vi "Adjustmentlog.vi"(5 "Variant":string, 7 "nominalLevel":string, 8 "error in (no error)":errorcluster, 9 "Level":dbl[](array[numeric]), 10 "Amplitude":dbl[](array[numeric]), 11 "Frequencies":dbl[](array[numeric])) -> (0 "error IO":errorcluster)   [LabVIEW 2018]
panel:
  out "concatenated string":string caption="File Content"
  out "date/time string":string
  out "path":path
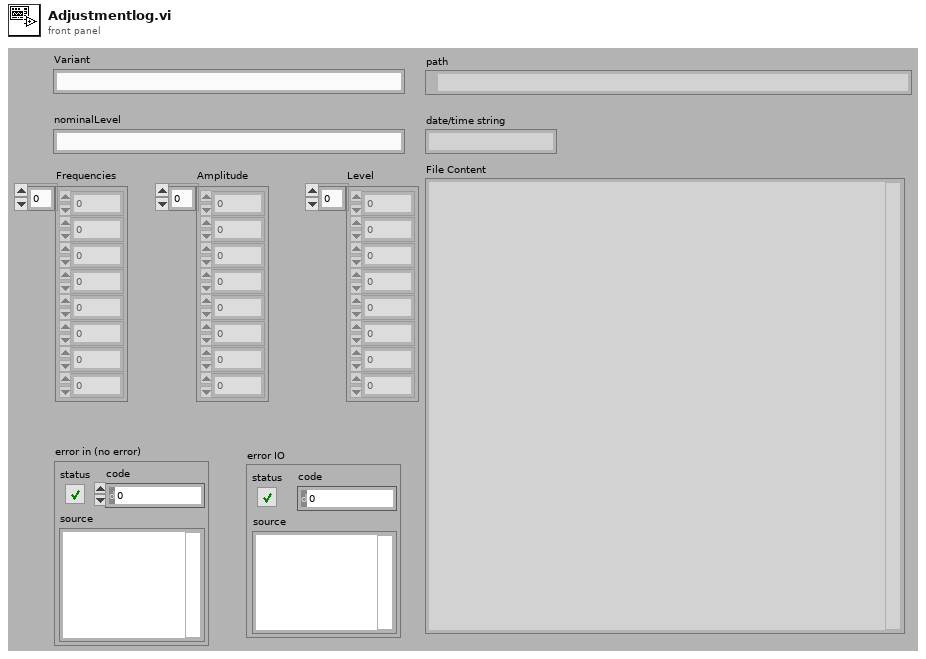
[diagram p1: front panel]
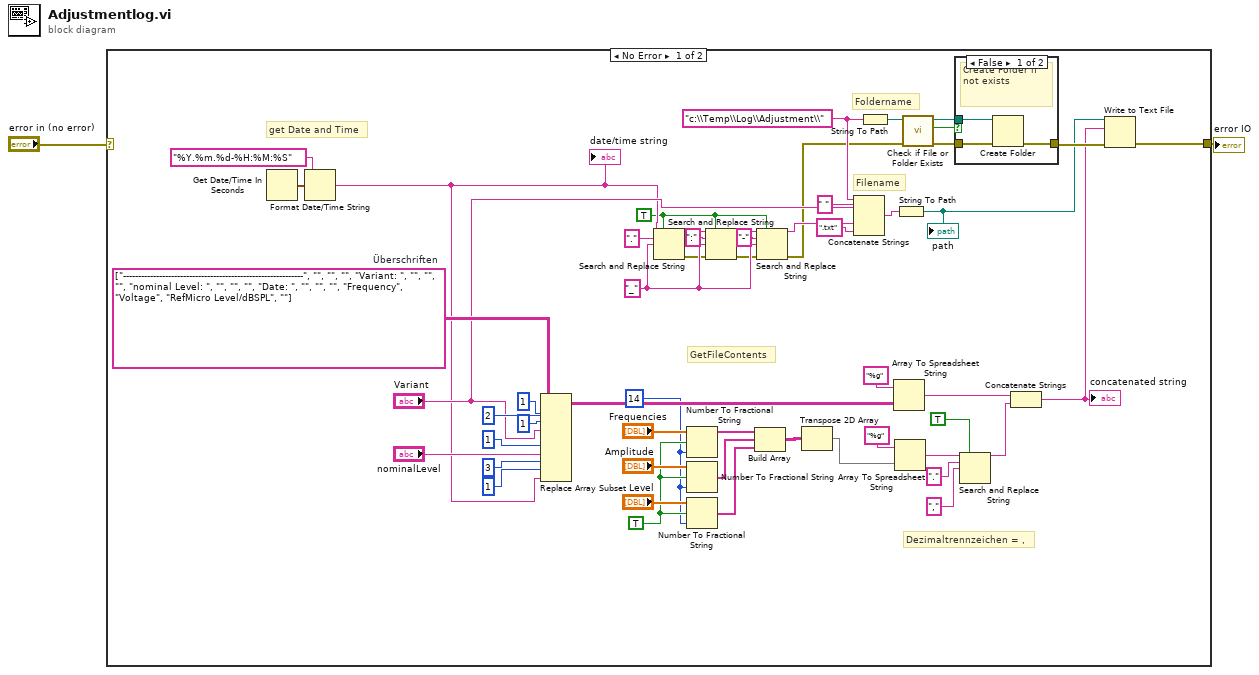
[diagram p0: block diagram]
diagram:
  n1 = case shown="No Error" "error in (no error)" {
    selector: "error in (no error)" -> [_ w61]
    tunnel: [w53 w61] -> w2
    frame No Error {
      w3 = i16 14 ("precision (6)")
      w5 = TRUE ("use system decimal point (T)")
      w34 = "_" ("replace string (\"\")")
      w31 = TRUE ("replace all? (F)")
      w25 = "c:\\Temp\\Log\\Adjustment\\" ("string")
      w46 = string[][] [["------------------------------------------------------------", "", "", ""], ["Variant: ", "", "", ""], ["nominal Level: ", "", "", ""], ["Date: ", "", "", ""], ["Frequency", "Voltage", "RefMicro Level/dBSPL", ""]]  # Überschriften
      # "Dezimaltrennzeichen = ,"
      # "get Date and Time"
      # "GetFileContents"
      # "Foldername"
      # "Filename"
      n2 = Get Date/Time In Seconds() -> (seconds since 1Jan1904=w43:timestamp)
      n3 = Format Date/Time String(time format string (%c)="%Y.%m.%d-%H:%M:%S", seconds (now)=w43) -> (date/time string=w38:string)  [unwired: 1 in]
      "date/time string" <- w38
      n4 = Replace Array Subset(array=w46, new element #1="Variant", index (row) #1=1 ("Index (Zeile)"), index (col) #1=1 ("Deaktivierter Index (Spalte)"), new element #2="nominalLevel", index (row) #2=2 ("Index (Zeile)"), index (col) #2=1 ("Deaktivierter Index (Spalte)"), new element #3=w38, index (row) #3=3 ("Index (Zeile)"), index (col) #3=1 ("Deaktivierter Index (Spalte)")) -> (w13:string[][])
      n5 = Search and Replace String(replace all?=w31, input string=w38, search string=".", replace string=w34) -> (result string=w36:string, error out=w22:errorcluster)  [unwired: 4 in, 2 out]
      n6 = Number To Fractional String(use system decimal point (T)=w5, number="Frequencies", precision (6)=w3) -> (F-format string=w19:string[])  [unwired: 1 in]
      n7 = Number To Fractional String(use system decimal point (T)=w5, number="Amplitude", precision (6)=w3) -> (F-format string=w54:string[])  [unwired: 1 in]
      n8 = Number To Fractional String(use system decimal point (T)=w5, number="Level", precision (6)=w3) -> (F-format string=w16:string[])  [unwired: 1 in]
      n9 = Search and Replace String(replace all?=w31, input string=w36, search string=":", replace string=w34, error in=w22) -> (result string=w35:string, error out=w21:errorcluster)  [unwired: 3 in, 2 out]
      n10 = Build Array(w19, w54, w16) -> (w45:string[][])
      n11 = Search and Replace String(replace all?=w31, input string=w35, search string="-", replace string=w34, error in=w21) -> (result string=w30:string, error out=w20:errorcluster)  [unwired: 3 in, 2 out]
      n12 = Transpose 2D Array(2D array=w45) -> (transposed array=w12:string[][])
      n13 = Concatenate Strings(w25, "Variant", " " ("string"), w30, ".txt" ("string")) -> (w39:string)
      n14 = String To Path(string=w25) -> (path=w24:path)
      n15 = Array To Spreadsheet String(array=w13, 3:"%g" ("Format-String")) -> (spreadsheet string=w6:string)  [unwired: 1 in]
      n16 = Array To Spreadsheet String(array=w12, 3:"%g" ("Format-String")) -> (spreadsheet string=w11:string)  [unwired: 1 in]
      n17 = String To Path(string=w39) -> (path=w23:path)
      "path" <- w23
      n18 = call <vilib>:"Check if File or Folder Exists.vi"("error in (no error)"=w20, "path"=w24) -> ("error out"=w29:errorcluster, "file or folder exists?"=w27:bool, "dup path"=w26:path)  [unwired: 7 in]
      n19 = case shown="False" w27 {
        tunnel: w29 -> [w59 w60]
        tunnel: [w58 w60] -> w28
        tunnel: w26 -> [w57 _]
        frame False {
          # "Create Folder if not exists"
          n20 = Create Folder(path (use dialog)=w57, error in=w59) -> (error out=w58:errorcluster)  [unwired: 1 in, 2 out]
        }
        frame True {
        }
      }
      n21 = Search and Replace String(replace all?=TRUE ("replace all? (F)"), input string=w11, search string="." ("."), replace string="," ("replace string (\"\")")) -> (result string=w7:string)  [unwired: 4 in, 3 out]
      n22 = Concatenate Strings(w6, w7) -> (w4:string)
      "concatenated string" <- w4
      n23 = Write to Text File(file (use dialog)=w23, text=w4, error in=w28) -> (error out=w53:errorcluster)  [unwired: 1 in, 2 out]
    }
    frame Error {
    }
  }
  "error IO" <- w2
